vi "Get USB Port.vi"(8 "Error In":errorcluster, 11 "object in":refnum<class "IConfigureViaUSB.lvclass">) -> (0 "Error Out":errorcluster, 2 "USB Port":string, 3 "object out":refnum<class "IConfigureViaUSB.lvclass">)   [LabVIEW 2023, in "IConfigureViaUSB.lvclass"]
uses:
  IConfigureViaUSB.lvclass
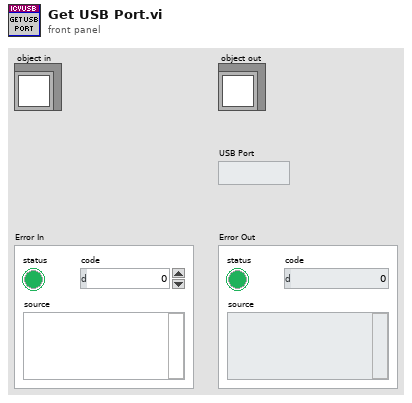
[diagram p1: front panel]
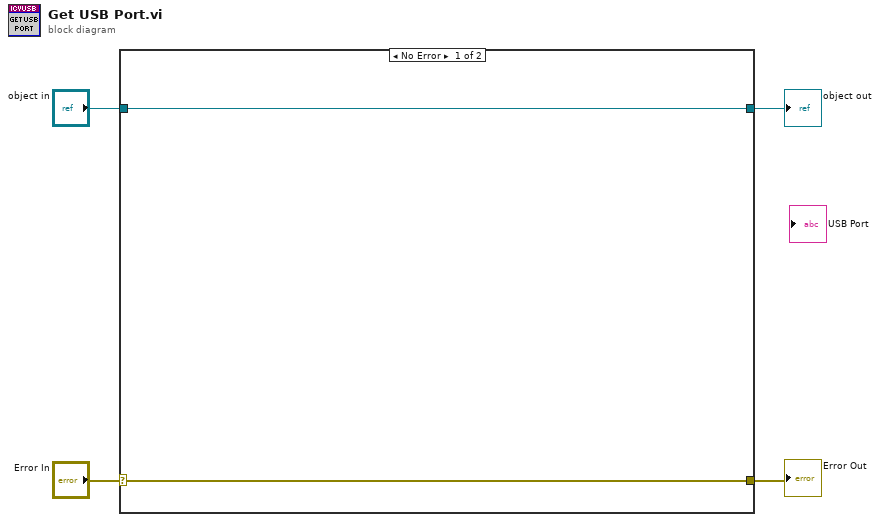
[diagram p0: block diagram]
diagram:
  n1 = case shown="No Error" "Error In" {
    selector: "Error In" -> [w6 w8]
    tunnel: [w6 w8] -> w3
    tunnel: [w5 w7] -> w1
    tunnel: "object in" -> [w5 w7]
    frame No Error {
    }
    frame Error {
    }
  }
  "Error Out" <- w3
  "object out" <- w1
